vi "Scan Instrument Info.vi"(0 "VISA resource name":refnum<visa-resource-name>, 1 "ID String in":string, 2 "Private.VI Refnum":T1) -> (4 "Manufacturer":string, 5 "Revision":string, 6 "VISA resource name Out":refnum<visa-resource-name>, 7 "Model":string, 8 "Info":string, 9 "error out":errorcluster)   [LabVIEW 2020]
uses:
  Sub Controls/Instrument Ref.ctl
  Sub Controls/Scan Output.ctl
  Sub Controls/Instrument Actions.ctl
  <vilib>/regexp/Match Regular Expression.xnode
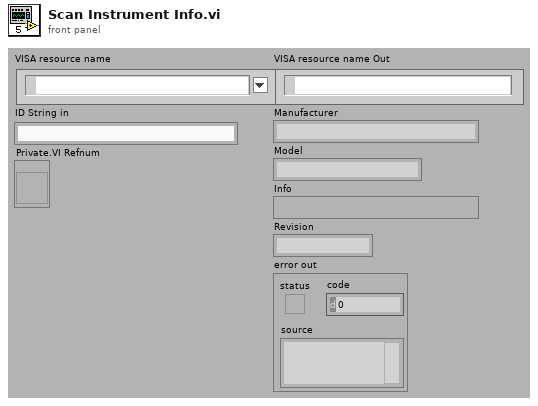
[diagram p1: front panel]
types:
  T1 = typedef "Instrument Ref.ctl" = refnum<vi>
  T2 = typedef "Instrument Actions.ctl" = enum16{"Scan", "Identify", "New", "Configure", "Initialize", "Test", "Read", "Close"}
  T3 = typedef "Scan Output.ctl" = cluster{"Manufacturer":string, "Model":string, "Info":string, "Revision":string, "error out":errorcluster}
  T4 = cluster{"VISA resource name":refnum<visa-resource-name>, "ID String in":string}
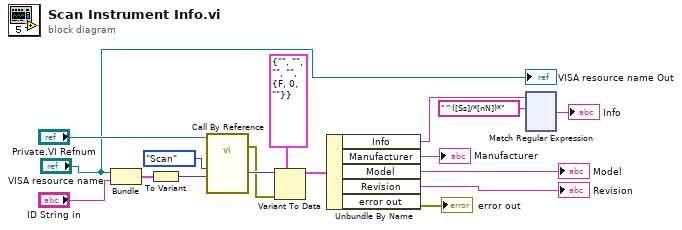
[diagram p0: block diagram]
diagram:
  n1 = Bundle("VISA resource name"="VISA resource name", "ID String in"="ID String in") -> (w15:T4)  [unwired: 1 in]
  n2 = To Variant(anything=w15) -> (Variant=w14:variant)
  n3 = call-by-ref "Call By Reference"(reference="Private.VI Refnum", "Action"=Instrument_Actions."Scan", "Parameters"=w14) -> (error out=w5:errorcluster, "Output"=w13:variant)  [unwired: 5 in, 2 out]
  n4 = Variant To Data(error in=w5, type=T3 {"Manufacturer"="", "Model"="", "Info"="", "Revision"="", "error out"={"status"=FALSE, "code"=0, "source"=""}} ("Scan Output"), Variant=w13) -> (data=w11:T3)  [unwired: 1 out]
  n5 = Unbundle By Name(w11) -> ("Info"=w2:string, "Manufacturer"=→"Manufacturer":string, "Model"=→"Model":string, "Revision"=→"Revision":string, "error out"=→"error out":errorcluster)
  n6 = xnode "Match Regular Expression"("input string"=w2, "regular expression"="^([Ss]/*[nN])*") -> ("after match"=→"Info":string)  [unwired: 4 in, 4 out]
  "VISA resource name Out" <- "VISA resource name"
